vi "A scan.vi"(4 "Channel name":string="0", 5 "Trigger level":dbl=2.0 format="%.2f", 6 "Min record length":i32=150 caption="Record length", 7 "Trigger delay":dbl=9.260000000000001e-06 format="%.3p", 8 "Min sample rate":dbl=500000000.0 caption="Sample rate" format="%.2p", 9 "Vertical range":dbl=0.25 format="%.2f", 10 "Trigger source":T1="VAL_EXTERNAL", 11 "Resource name":refnum<k15>="PXI1Slot5" caption="DAQ") -> (0 "Signal":waveform(dbl)[](array[waveform]), 1 "Error out":errorcluster caption="error out", 2 "Instrument handle out":refnum<k15>, 3 "A-SCAN":dbl[][](graph)=[[0.005187187576666474, 0.0, -0.003458125051110983, -0.0017290625255554914, 0.0, 0.0, 0.0, -0.0017290625255554914, 0.0, 0.0, 0.0, 0.0, -0.0017290625255554914, -0.0017290625255554914, 0.0, 0.0017290625255554914, 0.0, -0.003458125051110983, -0.0017290625255554914, -0.0017290625255554914, 0.0, 0.0, 0.0, 0.0017290625255554914, 0.0017290625255554914, 0.0, -0.0017290625255554914, -0.0017290625255554914, 0.0017290625255554914, 0.0017290625255554914, 0.0017290625255554914, -0.0017290625255554914, -0.003458125051110983, -0.0017290625255554914, 0.0, -0.0017290625255554914, -0.0017290625255554914, -0.0017290625255554914, 0.0, 0.0, -0.003458125051110983, 0.0, 0.0017290625255554914, -0.0017290625255554914, -0.0017290625255554914, 0.0, 0.003458125051110983, 0.0017290625255554914, -0.0017290625255554914, -0.0017290625255554914, 0.0, 0.0, 0.0, -0.0017290625255554914, -0.0017290625255554914, -0.003458125051110983, -0.005187187576666474, -0.0017290625255554914, 0.02593593788333237, 0.04668468818999827, 0.017290625255554914, -0.05878812586888671, -0.09509843890555203, -0.03631031303666532, 0.055330000817775726, 0.07607875112444162, 0.02420687535777688, -0.015561562729999423, -0.008645312627777457, 0.005187187576666474, -0.005187187576666474, -0.01210343767888844, -0.005187187576666474, 0.0, 0.0, -0.0017290625255554914, 0.0, 0.0, -0.0017290625255554914, 0.0, 0.0, 0.0, -0.0017290625255554914, -0.0017290625255554914, 0.0, 0.0, 0.0, -0.0017290625255554914, -0.0017290625255554914, -0.003458125051110983, -0.003458125051110983, 0.0, 0.0, -0.003458125051110983, -0.0017290625255554914, -0.0017290625255554914, -0.0017290625255554914, 0.0, -0.0017290625255554914, -0.0017290625255554914, 0.0017290625255554914, 0.0017290625255554914, 0.0017290625255554914, 0.005187187576666474, 0.0, -0.010374375153332949, -0.01210343767888844, -0.0017290625255554914, 0.005187187576666474, 0.003458125051110983, 0.0017290625255554914, 0.0017290625255554914, 0.003458125051110983, 0.003458125051110983, 0.0, 0.0, 0.0, -0.003458125051110983, 0.0, 0.0017290625255554914, 0.0017290625255554914, -0.003458125051110983, -0.0017290625255554914, -0.0017290625255554914, 0.0017290625255554914, 0.0017290625255554914, 0.0, -0.0017290625255554914, -0.0017290625255554914, 0.0, 0.0, 0.0, -0.0017290625255554914, -0.003458125051110983, 0.0, 0.003458125051110983, 0.0, 0.0, 0.0017290625255554914, 0.0017290625255554914, 0.0, -0.0017290625255554914, 0.0017290625255554914, 0.0017290625255554914, -0.003458125051110983, -0.005187187576666474, -0.005187187576666474, -0.003458125051110983, 0.0, 0.0]])   [LabVIEW 2014]
uses:
  <instrlib>/niScope/Controls/niScope trigger source.ctl
  <instrlib>/niScope/Controls/niScope trigger slope.ctl
  <instrlib>/niScope/Controls/niScope trigger coupling.ctl
  <instrlib>/niScope/Configure/Trigger/niScope Configure Trigger Edge.vi
  <instrlib>/niScope/Acquire/Fetch/niScope Multi Fetch WDT.vi
  <instrlib>/niScope/Acquire/Fetch/niScope Multi Fetch.vi
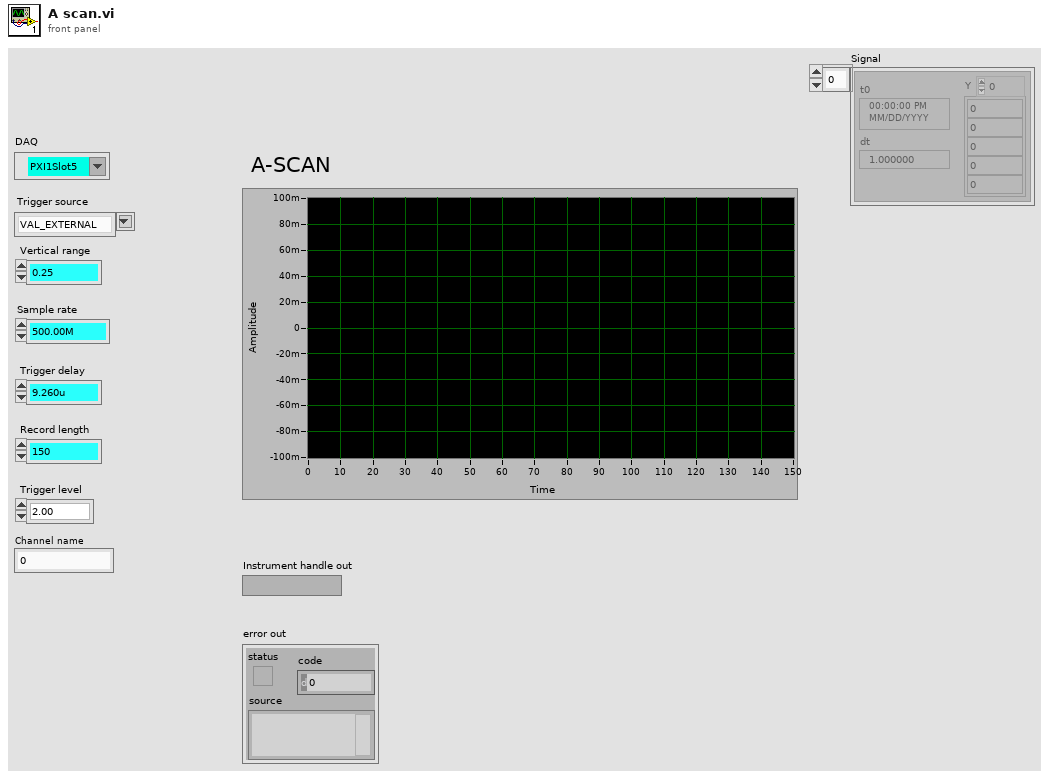
[diagram p1: front panel]
types:
  T1 = typedef "niScope trigger source.ctl" = string
  T2 = typedef "niScope trigger coupling.ctl" = u16
  T3 = typedef "niScope trigger slope.ctl" = i32
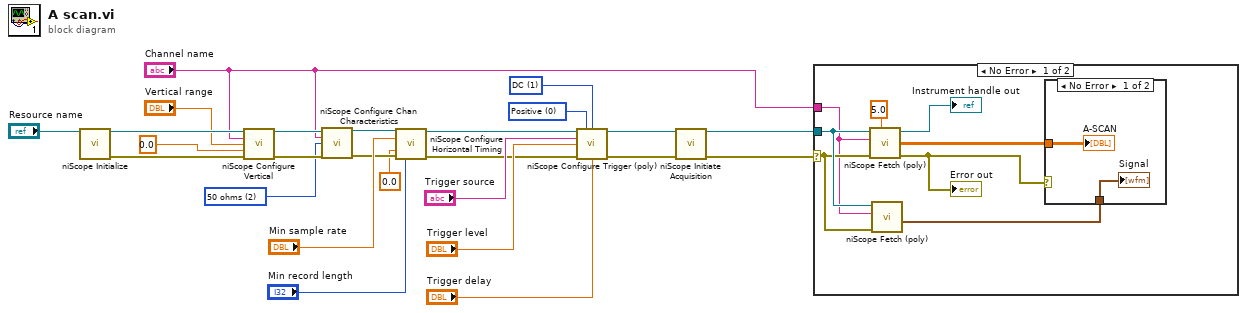
[diagram p0: block diagram]
diagram:
  w4 = T2 1 items=["AC"=0, "DC"=1, "HF Reject"=3, "LF Reject"=4, "AC Plus HF Reject"=1001] ("trigger coupling")
  w5 = T3 0 items=["Positive", "Negative"] ("trigger slope")
  w7 = u32 2 items=["1 mega ohm"=0, "50 ohms"=2] ("input impedance")
  n1 = call <instrlib>:"niScope Initialize.vi"("resource name"="Resource name") -> ("instrument handle"=w24:refnum<k15>, "error out"=w25:errorcluster)  [unwired: 13 in]
  n2 = call <instrlib>:"niScope Configure Vertical.vi"("instrument handle"=w24, "channels"="Channel name", "vertical range"="Vertical range", "vertical offset"=0.0, "error in"=w25) -> ("instrument handle out"=w15:refnum<k15>, "error out"=w13:errorcluster)  [unwired: 9 in]
  n3 = call <instrlib>:"niScope Configure Chan Characteristics.vi"("instrument handle"=w15, "channels"="Channel name", "input impedance"=w7, "error in"=w13) -> ("instrument handle out"=w16:refnum<k15>, "error out"=w14:errorcluster)  [unwired: 10 in]
  n4 = call <instrlib>:"niScope Configure Horizontal Timing.vi"("instrument handle"=w16, "min sample rate"="Min sample rate", "reference position"=0.0, "error in"=w14, "min record length"="Min record length") -> ("instrument handle out"=w12:refnum<k15>, "error out"=w11:errorcluster)  [unwired: 9 in]
  n5 = call-poly <instrlib>:"niScope Configure Trigger (poly).vi"("instrument handle"=w12, "trigger slope"=w5, "trigger coupling"=w4, "trigger source"="Trigger source", "trigger level"="Trigger level", "error in"=w11, "trigger delay"="Trigger delay") -> ("instrument handle out"=w9:refnum<k15>, "error out"=w10:errorcluster)  [unwired: 7 in]
  n6 = call <instrlib>:"niScope Initiate Acquisition.vi"("instrument handle"=w9, "error in"=w10) -> ("instrument handle out"=w2:refnum<k15>, "error out"=w3:errorcluster)  [unwired: 12 in]
  n7 = case shown="No Error" w3 {
    selector: w3 -> [w28 _]
    tunnel: w2 -> [w29 _]
    tunnel: "Channel name" -> [w26 _]
    frame No Error {
      n8 = call-poly <instrlib>:"niScope Fetch (poly).vi"("timeout"=5.0, "error in"=w28, "channels"=w26, "instrument handle"=w29) -> ("error out"=w31:errorcluster, "wfm"=w30:dbl[][], "instrument handle out"=→"Instrument handle out":refnum<k15>)  [unwired: 4 in, 1 out]
      "Error out" <- w31
      n9 = call-poly <instrlib>:"niScope Fetch (poly).vi"("error in"=w28, "channels"=w26, "instrument handle"=w29) -> ("wfm"=w27:waveform(dbl)[])  [unwired: 5 in, 3 out]
      n10 = case shown="No Error" w31 {
        tunnel: w30 -> [w35 _]
        tunnel: w27 -> [w34 _]
        frame No Error {
          "A-SCAN" <- w35
          "Signal" <- w34
        }
        frame Error {
        }
      }
    }
    frame Error {
    }
  }
